vi "SimpleSetUpAcqu.vi"() -> ()   [LabVIEW 2011]
uses:
  <vilib>/Platform/TimedLoop/XDataNode/timing_clust.ctl
  <vilib>/Platform/TimedLoop/XDataNode/nitl_modes.ctl
  <vilib>/Platform/TimedLoop/XDataNode/wakeup.ctl
  Basler - A504 Comm tool.llb/1301_BASLER_A504_TD_commands.ctl
  <vilib>/Platform/TimedLoop/XDataNode/XDataNode.xnode
  <vilib>/Platform/TimedLoop/XDataNode/XDNodeRunTimeDep.lvlib
  <vilib>/ptbypt/NI_PtbyPt.lvlib
panel:
  in  "Stop":bool
  out "FPS":u32
  in  "Parameters":T1={"Frame rate"=100, "Exposure time"=160, "Trig?"=TRUE} {"Frame rate" max=100000 step=1}
  in  "Acquisition Window":T2={"Height"=128, "Left"=0, "Top"=0, "Width"=1000}
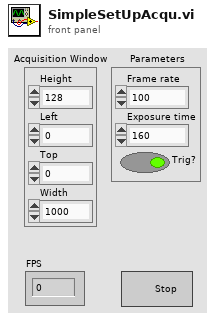
[diagram p1: front panel]
types:
  T1 = cluster{"Frame rate":u32, "Exposure time":u32, "Trig?":bool}
  T2 = cluster{"Height":u32, "Left":i32, "Top":u32, "Width":u32}
  T3 = typedef "1301_BASLER_A504_TD_commands.ctl" = enum16{"Read Status", "Exposer Time [us]", "Frame Rate", "ROI start column", "ROI width column", "ROI starting line", "ROI height in lines", "Free-Run", "ExSync programmable", "ExSync Level-controlled", "ExSync Edge-controlled", "Set Gain", "Set PosOffset", "Set NegOffset", "reset"}
  T4 = typedef "Image Type" = u32
  T5 = typedef "IMAQ Image.ctl" = refnum<image>
  T6 = typedef "XDNodeRunTimeDep.lvlib/timing_clust.ctl" = cluster{"Expected End [f-1]":u64, "Actual End [f-1]":u64, "Finished Late? [f-1]":bool, "Expected End [i-1]":u64, "Actual End [i-1]":u64, "Finished Late? [i-1]":bool, "Expected Start [i]":u64, "Actual Start [i]":u64, "Expected Start [f]":u64, "Actual Start [f]":u64, "Source Name":string, "Structure Name":string, "Period":i64, "Deadline":i64, "Offset":i64, "Start":i64, "Priority":i32, "Timeout":i32, "Mode":T7, "Wakeup Reason":T8, "Error":errorcluster, "Source Type":string, "Secondary Source Type":string, "Global End Time":u64, "Global Start Time":u64, "Frame Duration":u64, "Iteration Duration":u64, "Assigned CPU":i32, "I/O Scan Engine Mode":u32}
  T7 = typedef "XDNodeRunTimeDep.lvlib/nitl_modes.ctl" = enum32{"No Change", "Process missed periods, maintain original phase", "Discard missed periods, maintain original phase", "Process missed periods, ignore original phase", "Discard missed periods, ignore original phase"}
  T8 = typedef "XDNodeRunTimeDep.lvlib/wakeup.ctl" = enum32{"Normal", "Aborted", "Asynchronous wakeup", "Timing source error", "Timed loop error", "Timeout"}
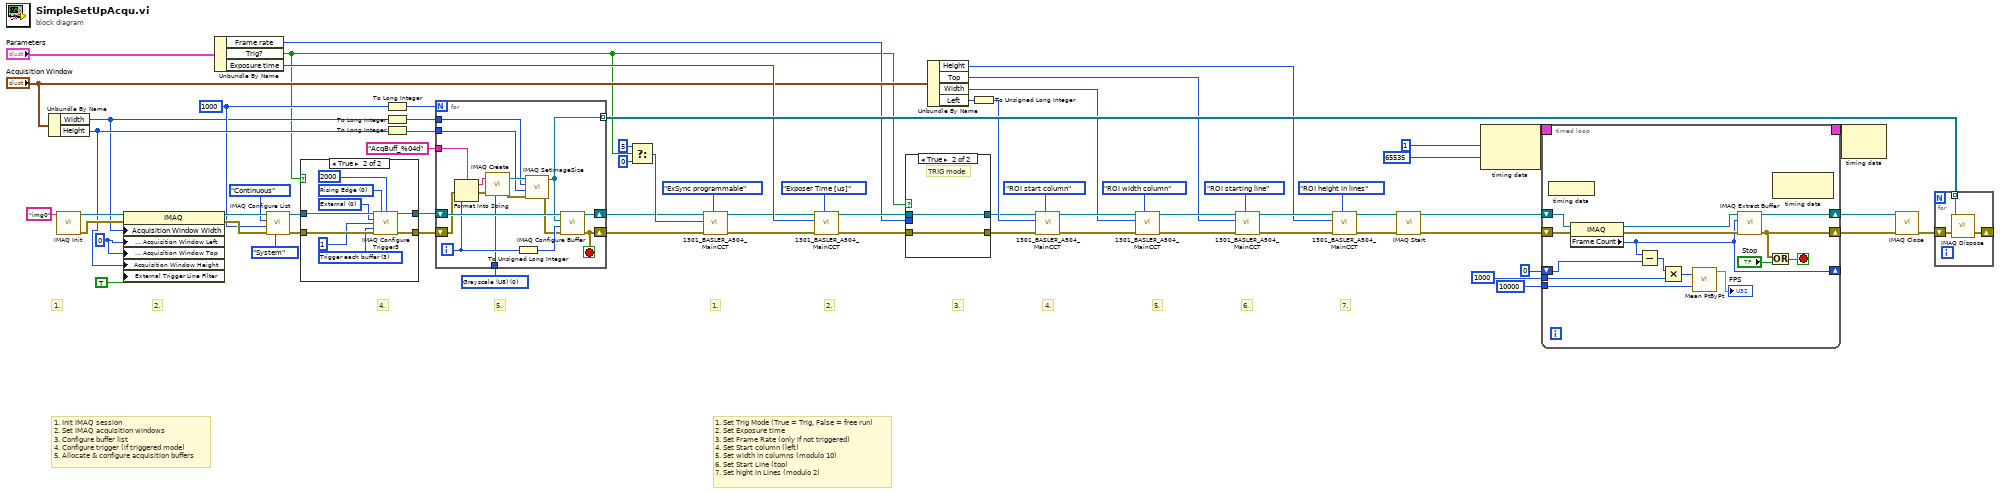
[diagram p0: block diagram]
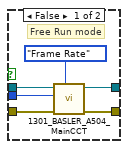
[diagram p2: hidden frame]
diagram:
  w45 = T4 0 items=["Grayscale (U8)", "Grayscale (I16)", "Grayscale (SGL)", "Complex (CSG)", "RGB (U32)", "HSL (U32)", "RGB (U64)", "Grayscale (U16)"] ("Image Type")
  w20 = u32 1000 ("Number of buffers")
  w52 = u32 0 ("Session Information : Acquisition Window Top")
  # "1."
  # "2."
  # "4."
  # "5."
  # "7."
  # "1. Init IMAQ session\n2. Set IMAQ acquisition windows\n3. Configure buffer list\n4. Configure trigger (if triggered mode)\n5. Allocate & configure acquisition buffers"
  # "1."
  # "2."
  # "3."
  # "4."
  # "5."
  # "6."
  # "1. Set Trig Mode (True = Trig, False = free run)\n2. Set Exposure time\n3. Set Frame Rate (only if not triggered)\n4. Set Start column (left)\n5. Set width in columns (modulo 10)\n6. Set Start Line (top)\n7. Set hight in Lines (modulo 2)"
  n1 = Unbundle By Name("Acquisition Window") -> ("Width"=w17:u32, "Height"=w22:u32)
  n2 = call <vilib>:"IMAQ Init.vi"("Interface Name"="img0") -> ("error out"=w44:errorcluster, "IMAQ Session Out"=w69:refnum<k11>)  [unwired: 9 in]
  n3 = property class="IMAQ"(reference=w69, error in=w44, "Acquisition Window Width"=w17, "Session Information : Acquisition Window Left"=w52, "Session Information : Acquisition Window Top"=w52, "Acquisition Window Height"=w22, "External Trigger Line Filter"=TRUE ("Acquisition Parameters : External Trigger Line Filter")) -> (reference out=w54:refnum<k11>, error out=w53:errorcluster)
  n4 = Unbundle By Name("Parameters") -> ("Frame rate"=w6:u32, "Trig?"=w5:bool, "Exposure time"=w43:u32)
  n5 = call <vilib>:"IMAQ Configure List.vi"("Memory Location"=enum16{"System", "Onboard"}."System", "error in (no error)"=w53, "Number of buffers"=w20, "Continuous?"=enum16{"One-Shot", "Continuous"}."Continuous", "IMAQ Session In"=w54) -> ("error out"=w51:errorcluster, "IMAQ Session Out"=w50:refnum<k11>)  [unwired: 5 in]
  n6 = case shown="True" w5 {
    tunnel: w51 -> [w70 w80]
    tunnel: w50 -> [w71 w79]
    tunnel: [w71 w78] -> w49
    tunnel: [w70 w77] -> w48
    frame False {
    }
    frame True {
      w72 = u32 3 items=["Disabled", "Trigger start of acquisition", "Trigger start of each buffer list", "Trigger each buffer", "Trigger each line (linescan)", "Trigger end of acquisition"] ("Action")
      w74 = u32 0 items=["External"=0, "RTSI"=1, "ISO In"=2, "Scaled Encoder"=5, "Software Trigger"=6] ("Type")
      w76 = u32 0 items=["Rising Edge", "Falling Edge"] ("Polarity")
      n7 = call <vilib>:"IMAQ Configure Trigger3.vi"("IMAQ Session In"=w79, "Polarity"=w76, "Frame timeout (ms)"=u32 2000, "Type"=w74, "Line Number"=u32 1, "Action"=w72, "error in (no error)"=w80) -> ("IMAQ Session Out"=w78:refnum<k11>, "error out"=w77:errorcluster)  [unwired: 2 in, 5 out]
    }
  }
  n8 = To Long Integer(number=w20) -> (32bit integer=w19:i32)
  n9 = To Long Integer(number=w17) -> (32bit integer=w23:i32)
  n10 = To Long Integer(number=w22) -> (32bit integer=w21:i32)
  n11 = for {
    N: w19 -> [_]
    shift-right: [w95] -> w14
    shift-left: w48 -> [w84]
    shift-right: [w93] -> w15
    shift-left: w49 -> [w94]
    tunnel: "AcqBuff_%04d" ("format string") -> [w91]
    tunnel: w45 -> [w88]
    tunnel: w23 -> [w82]
    tunnel: w21 -> [w81]
    tunnel: [w83] -> w57 mode=indexing
    i -> [w90]
    stop <- w95 stop-if-true
    n12 = Format Into String(format string=w91, error in=w84, w90) -> (resulting string=w92:string, error out=w87:errorcluster)  [unwired: 1 in]
    n13 = call "IMAQ Create"("Image Name"=w92, "Image Type"=w88, "error in (no error)"=w87) -> ("New Image"=w89:T5, "error out"=w86:errorcluster)  [unwired: 2 in]
    n14 = To Unsigned Long Integer(number=w90) -> (unsigned 32bit integer=w96:u32)
    n15 = call "IMAQ SetImageSize"("error in (no error)"=w86, "Y Resolution"=w81, "X Resolution"=w82, "Image"=w89) -> ("error out"=w85:errorcluster, "Image Out"=w83:T5)  [unwired: 1 in]
    n16 = call <vilib>:"IMAQ Configure Buffer.vi"("error in (no error)"=w85, "Buffer Number"=w96, "Image In"=w83, "IMAQ Session In"=w94) -> ("error out"=w95:errorcluster, "IMAQ Session Out"=w93:refnum<k11>)  [unwired: 6 in]
  }
  n17 = Select(t=u32 5, s=w5, f=u32 0) -> (s? t:f=w36:u32)
  n18 = call "1301_BASLER_A504_MainCCT.vi"("Commands"=1301_BASLER_A504_TD_commands."ExSync programmable", "error in"=w14, "Parameter"=w36, "Session In"=w15) -> ("error out"=w13:errorcluster, "Session out"=w12:refnum<k11>)  [unwired: 5 in, 1 out]
  n19 = call "1301_BASLER_A504_MainCCT.vi"("Commands"=1301_BASLER_A504_TD_commands."Exposer Time [us]", "error in"=w13, "Parameter"=w43, "Session In"=w12) -> ("error out"=w9:errorcluster, "Session out"=w8:refnum<k11>)  [unwired: 5 in, 1 out]
  n20 = case shown="True" w5 {
    tunnel: w9 -> [w101 w103]
    tunnel: w8 -> [w100 w104]
    tunnel: [w99 w104] -> w7
    tunnel: w6 -> [w98 _]
    tunnel: [w97 w103] -> w4
    frame False {
      # "Free Run mode"
      n21 = call "1301_BASLER_A504_MainCCT.vi"("Commands"=1301_BASLER_A504_TD_commands."Frame Rate", "error in"=w101, "Parameter"=w98, "Session In"=w100) -> ("error out"=w97:errorcluster, "Session out"=w99:refnum<k11>)  [unwired: 5 in, 1 out]
    }
    frame True {
      # "TRIG mode"
    }
  }
  n22 = Unbundle By Name("Acquisition Window") -> ("Height"=w24:u32, "Top"=w25:u32, "Width"=w26:u32, "Left"=w27:i32)
  n23 = To Unsigned Long Integer(number=w27) -> (unsigned 32bit integer=w18:u32)
  n24 = call "1301_BASLER_A504_MainCCT.vi"("Commands"=1301_BASLER_A504_TD_commands."ROI start column", "error in"=w4, "Parameter"=w18, "Session In"=w7) -> ("error out"=w32:errorcluster, "Session out"=w29:refnum<k11>)  [unwired: 5 in, 1 out]
  n25 = call "1301_BASLER_A504_MainCCT.vi"("Commands"=1301_BASLER_A504_TD_commands."ROI width column", "error in"=w32, "Parameter"=w26, "Session In"=w29) -> ("error out"=w33:errorcluster, "Session out"=w30:refnum<k11>)  [unwired: 5 in, 1 out]
  n26 = call "1301_BASLER_A504_MainCCT.vi"("Commands"=1301_BASLER_A504_TD_commands."ROI starting line", "error in"=w33, "Parameter"=w25, "Session In"=w30) -> ("error out"=w34:errorcluster, "Session out"=w31:refnum<k11>)  [unwired: 5 in, 1 out]
  n27 = call "1301_BASLER_A504_MainCCT.vi"("Commands"=1301_BASLER_A504_TD_commands."ROI height in lines", "error in"=w34, "Parameter"=w24, "Session In"=w31) -> ("error out"=w10:errorcluster, "Session out"=w11:refnum<k11>)  [unwired: 5 in, 1 out]
  n28 = call <vilib>:"IMAQ Start.vi"("error in (no error)"=w10, "IMAQ Session In"=w11) -> ("error out"=w62:errorcluster, "IMAQ Session Out"=w64:refnum<k11>)  [unwired: 8 in]
  n29 = node-c288(i64 1 ("Period"), 65535 ("Priority")) -> (w66:T6)
  n30 = timed-loop {
    timing: w66 -> [_]
    timing-out: [_] -> w65
    shift-right: [w108] -> w63
    shift-left: w62 -> [w113]
    shift-right: [w111] -> w61
    shift-left: w64 -> [w112]
    shift-right: [w110] -> _
    shift-left: u32 0 ("Last Valid Frame") -> [w107]
    tunnel: u32 1000 ("y") -> [w106]
    tunnel: 10000 ("sample length") -> [w105]
    stop <- w109 stop-if-true
    n31 = node-c288() -> ()  [unwired: 1 in]
    n32 = property class="IMAQ"(reference=w112, error in=w113) -> (reference out=w118:refnum<k11>, error out=w117:errorcluster, "Frame Count"=w110:u32)
    n33 = Subtract(x=w110, y=w107) -> (x-y=w116:u32)
    n34 = Multiply(x=w116, y=w106) -> (x*y=w115:u32)
    n35 = call <vilib>:"Mean PtByPt.vi"("x"=w115, "sample length"=w105) -> ("mean"=→"FPS":dbl)  [unwired: 2 in, 1 out]
    n36 = call <vilib>:"IMAQ Extract Buffer.vi"("error in (no error)"=w117, "Buffer to extract"=w110, "IMAQ Session In"=w118) -> ("error out"=w108:errorcluster, "IMAQ Session Out"=w111:refnum<k11>)  [unwired: 3 in, 4 out]
    n37 = Or(x=w108, y="Stop") -> (x .or. y?=w109:bool)
    n38 = node-c288() -> ()  [unwired: 1 in, 1 out]
  }
  n39 = node-c288(w65) -> ()  [unwired: 1 out]
  n40 = call <vilib>:"IMAQ Close.vi"("error in (no error)"=w63, "IMAQ Session In"=w61) -> ("error out"=w58:errorcluster)  [unwired: 9 in]
  n41 = for {
    tunnel: w57 -> [w123] mode=indexing
    shift-right: [w122] -> _
    shift-left: w58 -> [w124]
    n42 = call "IMAQ Dispose"("Image"=w123, "error in (no error)"=w124) -> ("error out"=w122:errorcluster)  [unwired: 4 in]
  }
